vi "PQerrorMessage.vi"(8 "error in (no error)":errorcluster, 11 "conn":u64) -> (0 "error out":errorcluster, 1 "PQerrorMessage":string, 3 "conn_out":u64)   [LabVIEW 2019, in "libpqlv64.lvlib"]
doc: "Returns the error message most recently generated by an operation on the connection."
uses:
  libpqlv64.lvlib
  libpq.dll
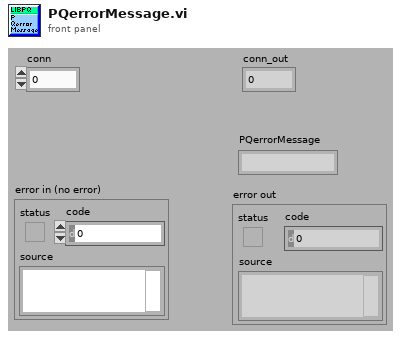
[diagram p1: front panel]
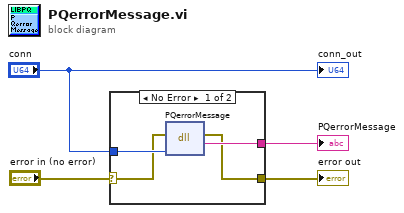
[diagram p0: block diagram]
diagram:
  n1 = case shown="No Error" "error in (no error)" {
    selector: "error in (no error)" -> [w6 w9]
    tunnel: [w5 w9] -> w3
    tunnel: [w8 _] -> w2
    tunnel: "conn" -> [w7 _]
    frame No Error {
      n2 = dll-call lib="libpq.*" fn="PQerrorMessage"(error in=w6, "conn"=w7) -> (error out=w5:errorcluster, "PQerrorMessage"=w8:string)  [unwired: 3 in, 1 out]
    }
    frame Error {
    }
  }
  "PQerrorMessage" <- w2
  "error out" <- w3
  "conn_out" <- "conn"
